vi "Assign DIO Bits For Jog Mode.vi"(4 "Axis (1)":i32=1 min=1 max=3, 5 "error in (no error)":errorcluster, 6 "Bit# in positive direction (0)":i32 min=0 max=15, 7 "Bit# in negative direction (0)":i32 min=0 max=15, 8 "VISA resource name":refnum<visa-resource-name>) -> (0 "error out":errorcluster, 3 "VISA resource name out":refnum<visa-resource-name>)   [LabVIEW 2019, in "Newport ESP301.lvlib"]
doc: "This command is used to assign DIO bits for jogging axes in either negative or positive directions."
uses:
  Newport ESP301.lvlib
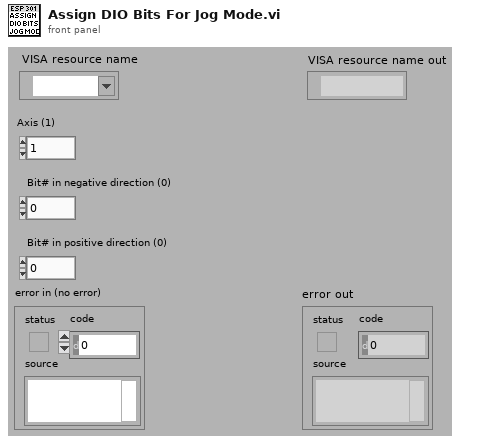
[diagram p1: front panel]
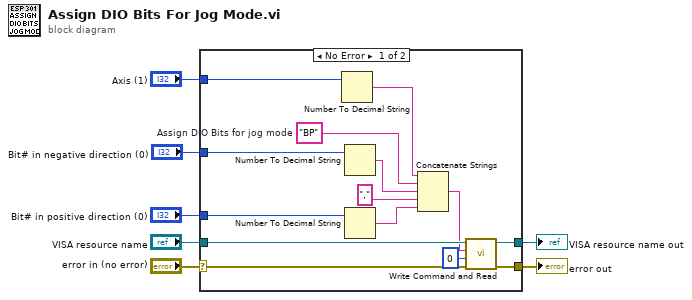
[diagram p0: block diagram]
diagram:
  n1 = case shown="No Error" "error in (no error)" {
    selector: "error in (no error)" -> [w20 w23]
    tunnel: [w19 w23] -> w7
    tunnel: "VISA resource name" -> [w21 w22]
    tunnel: [w18 w22] -> w6
    tunnel: "Axis (1)" -> [w15 _]
    tunnel: "Bit# in negative direction (0)" -> [w12 _]
    tunnel: "Bit# in positive direction (0)" -> [w8 _]
    frame No Error {
      w16 = "BP"  # Assign DIO Bits for jog mode
      n2 = Number To Decimal String(number=w15) -> (decimal integer string=w17:string)  [unwired: 1 out]
      n3 = Number To Decimal String(number=w12) -> (decimal integer string=w11:string)  [unwired: 1 out]
      n4 = Number To Decimal String(number=w8) -> (decimal integer string=w10:string)  [unwired: 1 out]
      n5 = Concatenate Strings(w17, w16, w11, "," ("Assign DIO Bits to Inhibit Motion"), w10) -> (w14:string)
      n6 = call "Write Command and Read.vi"("error in (no error)"=w20, "Bytes to read (100)"=u32 0, "Command"=w14, "VISA resource name"=w21) -> ("error out"=w19:errorcluster, "VISA resource name out"=w18:refnum<visa-resource-name>)  [unwired: 1 in, 3 out]
    }
    frame Error {
    }
  }
  "error out" <- w7
  "VISA resource name out" <- w6
